vi "usb relay init.vi"(8 "error in (no error)":errorcluster) -> (0 "error out":errorcluster, 3 "function return":i32)   [LabVIEW 2022 SP3, in "usb_relay_device.lvlib"]
doc: "int EXPORT_API usb_relay_init(void);"
uses:
  usb_relay_device.lvlib
  AppBuilderFiles/RunTimeExe/data/usb_relay_device.dll
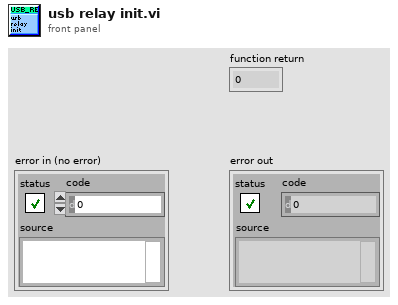
[diagram p1: front panel]
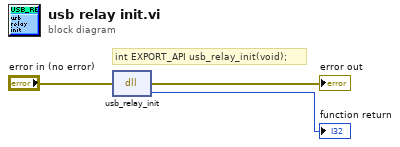
[diagram p0: block diagram]
diagram:
  # "int EXPORT_API usb_relay_init(void);"
  n1 = dll-call lib="D:/LabVIEWSuite_64_OS/AppBuilderFiles/RunTimeExe/data/usb_relay_device.*" fn="usb_relay_init"(error in="error in (no error)") -> (error out=→"error out":errorcluster, →"function return":i32)  [unwired: 2 in, 1 out]
